vi "Preprocess Commands.vi"(11 "Command In":T1={"Name"="", "CPTM.DataType"=variant, "All Control Values Variant"=[], "icon full"={"image type"=0, "image depth"=0, "image"=[], "mask"=[], "colors"=[], "Rectangle"={"left"=0, "top"=0, "right"=0, "bottom"=0}}, "icon scaled"={"image type"=0, "image depth"=0, "image"=[], "mask"=[], "colors"=[], "Rectangle"={"left"=0, "top"=0, "right"=0, "bottom"=0}}, "Path"=path "", "Subsystem Color"=16777216}) -> (3 "Command out":T3)   [LabVIEW 2025]
uses:
  bordeaux-2687-rebuilt/bordeaux-2687-rebuilt/Bordeaux/Types/Single Cmd Info.ctl
  <vilib>/picture/picture.llb/imagedata.ctl
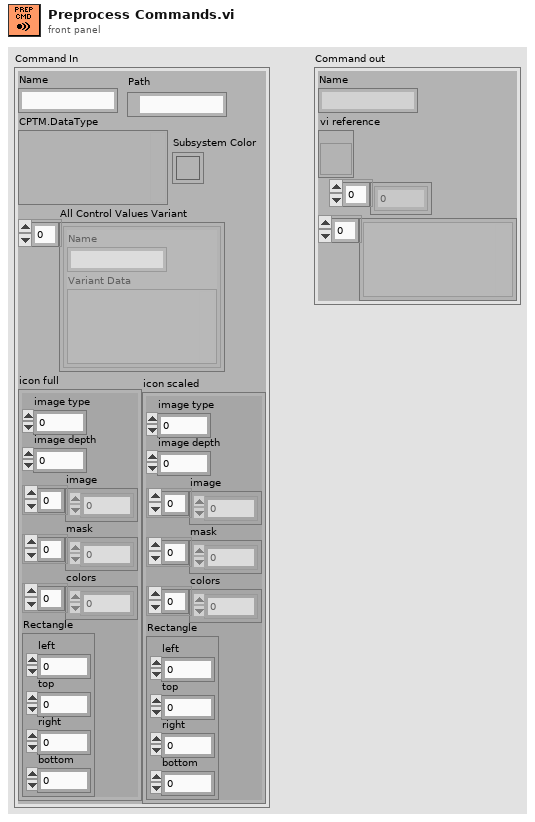
[diagram p1: front panel]
types:
  T1 = typedef "Single Cmd Info.ctl" = cluster{"Name":string, "CPTM.DataType":variant, "All Control Values Variant":cluster{"Name":string, "Variant Data":variant}[], "icon full":T2, "icon scaled":T2, "Path":path, "Subsystem Color":u32}
  T2 = typedef "imagedata.ctl" = cluster{"image type":i32, "image depth":i32, "image":u8[], "mask":u8[], "colors":u32[], "Rectangle":cluster{"left":i16, "top":i16, "right":i16, "bottom":i16}}
  T3 = cluster{"Name":string, "vi reference":refnum<vi>, i32[], variant[]}
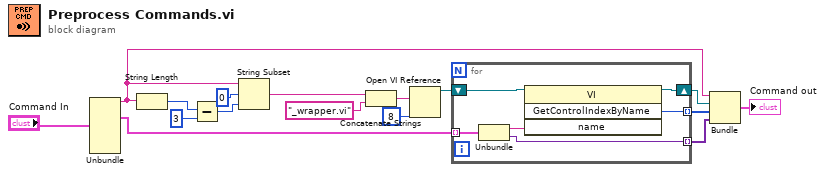
[diagram p0: block diagram]
diagram:
  n1 = Unbundle("Command In") -> ("Name"=w10:string, "All Control Values Variant"=w9:cluster{"Name":string, "Variant Data":variant}[])  [unwired: 5 out]
  n2 = String Length(string=w10) -> (length=w2:i32)
  n3 = Subtract(x=w2, y=3) -> (x-y=w3:i32)
  n4 = String Subset(string=w10, offset (0)=0, length (rest)=w3) -> (substring=w5:string)
  n5 = Concatenate Strings(w5, "_wrapper.vi" ("string")) -> (w7:string)
  n6 = Open VI Reference(vi path=w7, options=8) -> (vi reference=w8:refnum<vi>)  [unwired: 4 in, 1 out]
  n7 = for {
    tunnel: w9 -> [w20] mode=indexing
    shift-right: [w21] -> w11
    shift-left: w8 -> [w22]
    tunnel: [w18] -> w12 mode=indexing
    tunnel: [w17] -> w13 mode=indexing
    n8 = Unbundle(w20) -> ("Name"=w19:string, "Variant Data"=w17:variant)
    n9 = invoke class="VI" method="GetControlIndexByName"(reference=w22, "name"=w19) -> (reference out=w21:refnum<vi>, "GetControlIndexByName"=w18:i32)  [unwired: 2 in, 2 out]
  }
  n10 = Bundle("Name"=w10, "vi reference"=w11, w12, w13) -> (→"Command out":T3)  [unwired: 1 in]
